vi "Available Port.vi"() -> (1 "Available Port":u16)   [LabVIEW 2017]
doc: "Returns a UDP port number that the operating system reports as free for use."
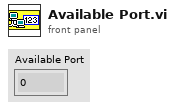
[diagram p1: front panel]
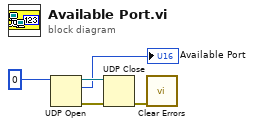
[diagram p0: block diagram]
diagram:
  n1 = UDP Open(11:u16 0 ("port")) -> (port=w4:refnum<k16>, 0:w5:errorcluster, 2:→"Available Port":u16)  [unwired: 4 in]
  n2 = UDP Close(connection ID=w4, 8:w5) -> (error out=w2:errorcluster)  [unwired: 1 out]
  n3 = call <vilib>:"Clear Errors.vi"("error in (no error)"=w2) -> ()  [unwired: 5 in, 2 out]
